vi "ArduinoDetectTram.vi"(3 "endChar":string=";", 4 "syncChar":string="@", 5 "bufferIN":string) -> (0 "dataDetected":bool, 1 "bufferOUT":string, 2 "data":string)   [LabVIEW 2024]
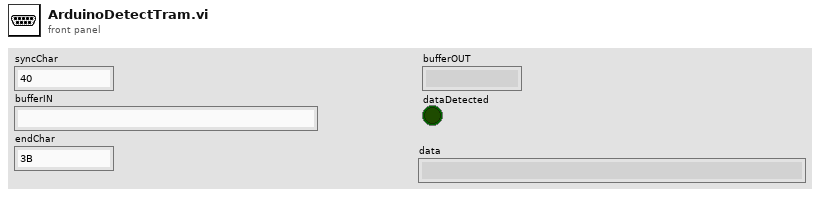
[diagram p1: front panel]
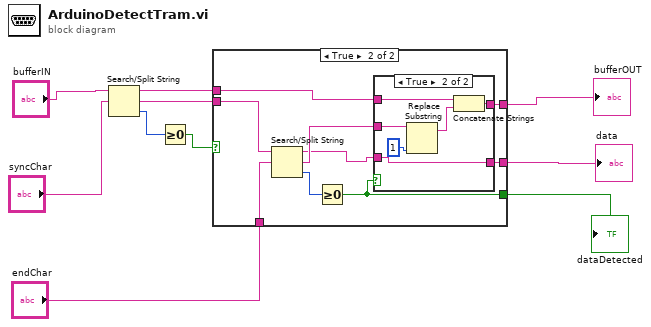
[diagram p0: block diagram]
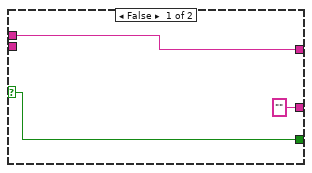
[diagram p2: hidden frame]
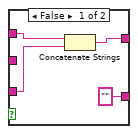
[diagram p3: hidden frame]
diagram:
  n1 = Search/Split String(string="bufferIN", search string/char (-)="syncChar") -> (substring before match=w10:string, match + rest of string=w9:string, offset of match=w8:i32)  [unwired: 1 in]
  n2 = Greater Or Equal To 0?(x=w8) -> (x >= 0?=w7:bool)
  n3 = case shown="True" w7 {
    selector: w7 -> [w13 _]
    tunnel: w9 -> [_ w21]
    tunnel: [w13 w17] -> w2
    tunnel: [w12 w20] -> w4
    tunnel: w10 -> [w12 w19]
    tunnel: ["" ("bufferRx") w15] -> w3
    tunnel: "endChar" -> [_ w14]
    frame False {
    }
    frame True {
      n4 = Search/Split String(string=w21, search string/char (-)=w14) -> (substring before match=w16:string, match + rest of string=w18:string, offset of match=w22:i32)  [unwired: 1 in]
      n5 = Greater Or Equal To 0?(x=w22) -> (x >= 0?=w17:bool)
      n6 = case shown="True" w17 {
        tunnel: [w24 w32] -> w20
        tunnel: w19 -> [w23 w31]
        tunnel: w18 -> [_ w30]
        tunnel: w16 -> [w26 w27]
        tunnel: ["" ("bufferRx") w27] -> w15
        frame False {
          n7 = Concatenate Strings(w23, w26) -> (w24:string)
        }
        frame True {
          n8 = Replace Substring(2:1 ("longueur (long. de la sous-chaîne)"), 5:w30) -> (1:w28:string)  [unwired: 2 in, 1 out]
          n9 = Concatenate Strings(w31, w28) -> (w32:string)
        }
      }
    }
  }
  "bufferOUT" <- w4
  "data" <- w3
  "dataDetected" <- w2
